vi "Enhance_No_of_points.vi"(3 "Enhancement factor":i32=2, 5 "Input":dbl[](array[numeric]) format="%.4f") -> (1 "Output":dbl[](array[numeric]) format="%.4f")   [LabVIEW 2010]
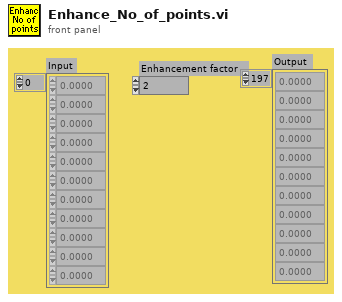
[diagram p1: front panel]
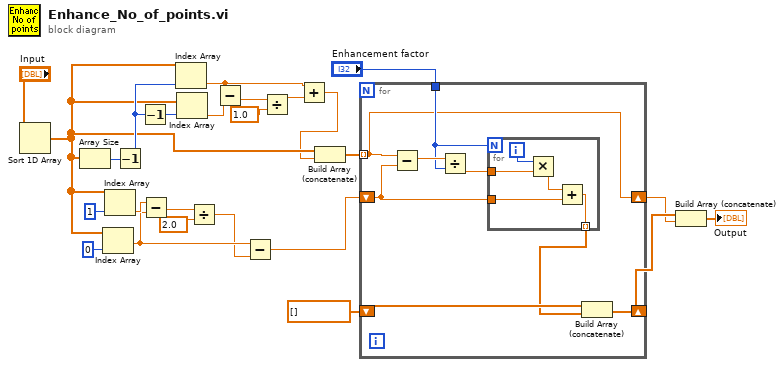
[diagram p0: block diagram]
diagram:
  n1 = Sort 1D Array(array="Input") -> (sorted array=w5:dbl[])
  n2 = Array Size(array=w5) -> (size(s)=w11:i32)
  n3 = Index Array(array=w5, index=0) -> (element=w16:dbl)
  n4 = Index Array(array=w5, index=1) -> (element=w17:dbl)
  n5 = Decrement(x=w11) -> (x-1=w10:i32)
  n6 = Decrement(x=w10) -> (x-1=w9:i32)
  n7 = Subtract(x=w17, y=w16) -> (x-y=w14:dbl)
  n8 = Index Array(array=w5, index=w10) -> (element=w2:dbl)
  n9 = Index Array(array=w5, index=w9) -> (element=w6:dbl)
  n10 = Divide(x=w14, y=2.0) -> (x/y=w12:dbl)
  n11 = Subtract(x=w2, y=w6) -> (x-y=w7:dbl)
  n12 = Subtract(x=w16, y=w12) -> (x-y=w15:dbl)
  n13 = Divide(x=w7, y=1.0) -> (x/y=w3:dbl)
  n14 = Add(x=w2, y=w3) -> (x+y=w1:dbl)
  n15 = Build Array (concatenate)(w5, w1) -> (w4:dbl[])
  n16 = for {
    shift-right: [w29] -> w20
    shift-left: w15 -> [w30]
    tunnel: w4 -> [w29] mode=indexing
    tunnel: "Enhancement factor" -> [w32]
    shift-right: [w28] -> w21
    shift-left: dbl[] [] -> [w27]
    n17 = Subtract(x=w29, y=w30) -> (x-y=w33:dbl)
    n18 = Divide(x=w33, y=w32) -> (x/y=w31:dbl)
    n19 = for {
      N: w32 -> [_]
      tunnel: w31 -> [w37]
      tunnel: w30 -> [w35]
      tunnel: [w34] -> w26 mode=indexing
      i -> [w38]
      n20 = Multiply(x=w38, y=w37) -> (x*y=w36:dbl)
      n21 = Add(x=w36, y=w35) -> (x+y=w34:dbl)
    }
    n22 = Build Array (concatenate)(w27, w26) -> (w28:dbl[])
  }
  n23 = Build Array (concatenate)(w21, w20) -> (→"Output":dbl[])
